vi "nivi.vi"() -> ()   [LabVIEW 2014]
uses:
  <vilib>/Analysis/NI_AALPro.lvlib
panel:
  in  "frequency 4":dbl=10.0 format="%0.2f"
  in  "frequency 3":dbl=10.0 format="%0.2f"
  out "unipolar NRZ 2":dbl[](graph)
  in  "frequency 2":dbl=10.0 format="%0.2f"
  in  "frequency":dbl=10.0 format="%0.2f"
  out "unipolar NRZ":dbl[](graph)
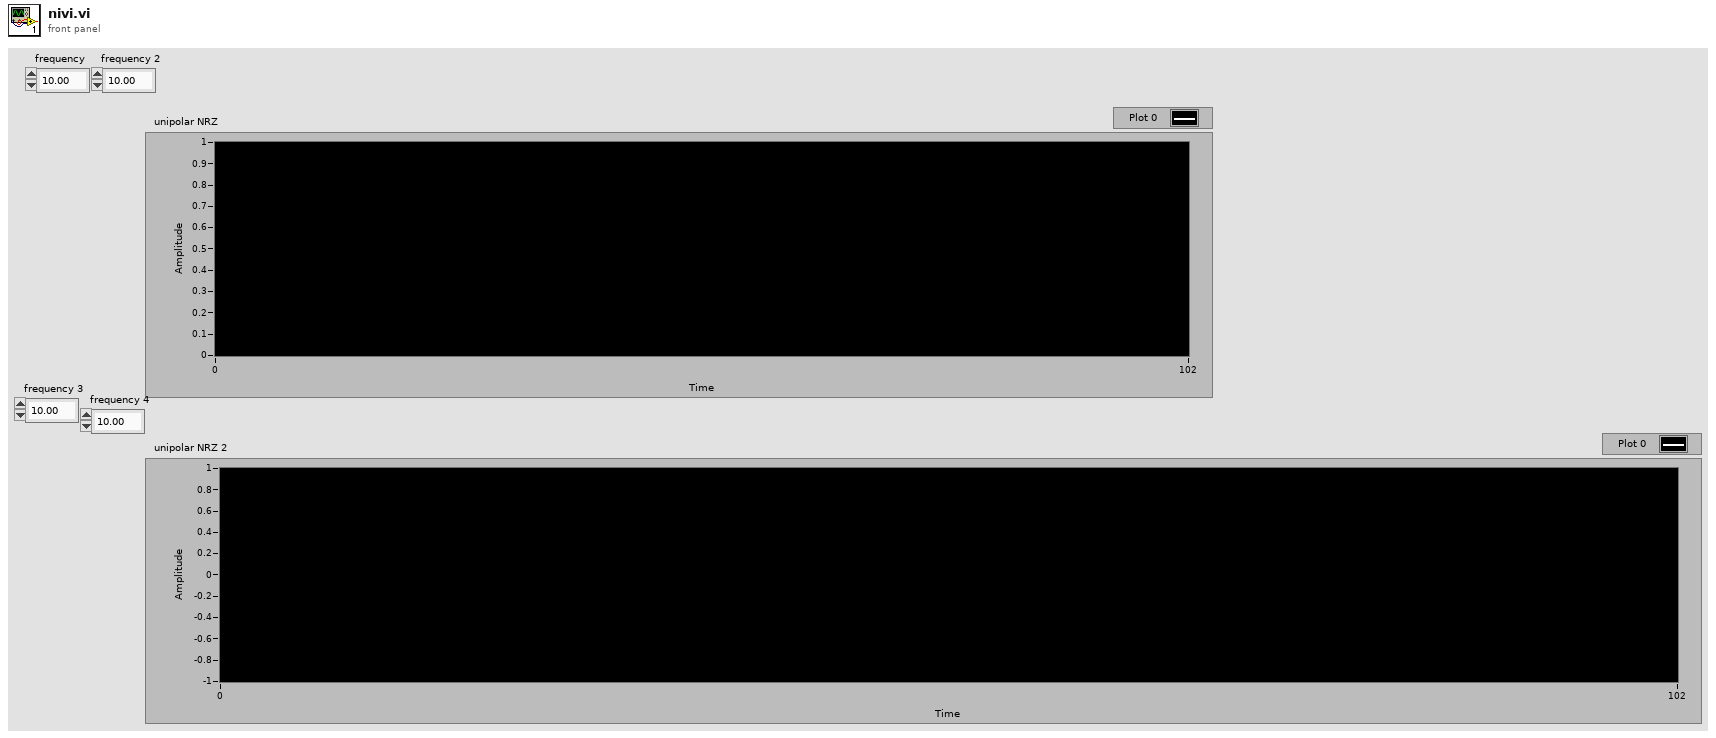
[diagram p1: front panel]
types:
  T1 = enum16{"sine", "cosine", "triangle", "square", "sawtooth", "increasing ramp", "decreasing ramp"}
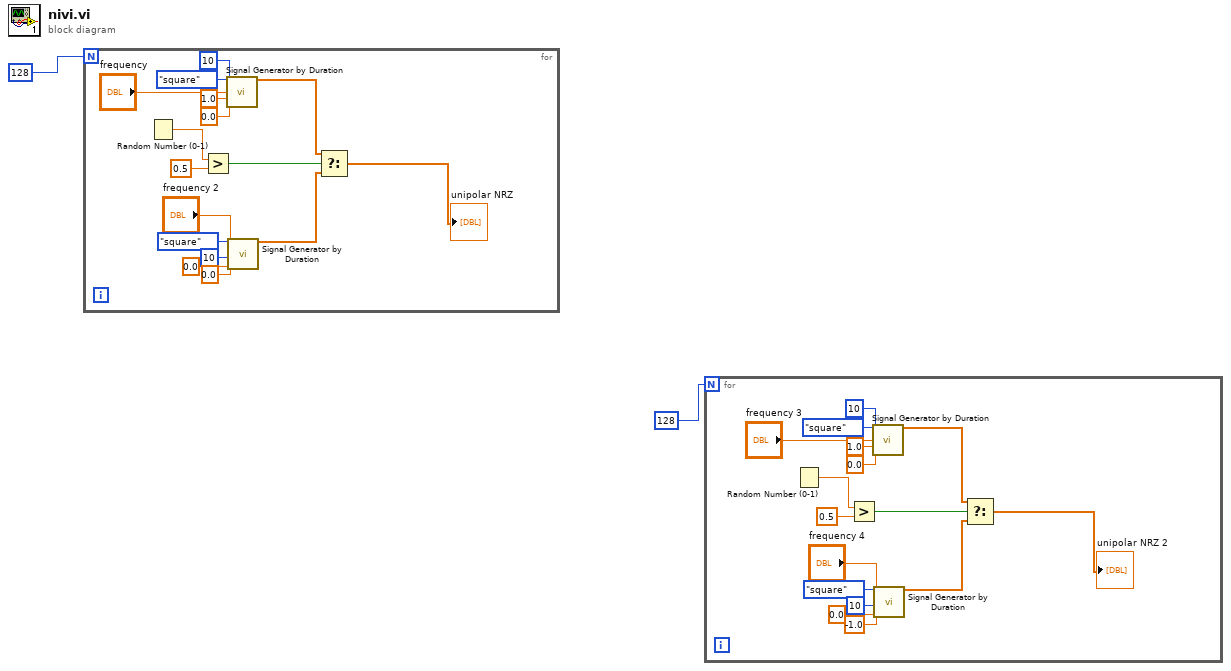
[diagram p0: block diagram]
diagram:
  n1 = for {
    N: 128 -> [_]
    n2 = Random Number (0-1)() -> (number: 0 to 1=w18:dbl)
    n3 = Greater?(x=w18, y=0.5) -> (0:w16:bool)
    n4 = call <vilib>:"Signal Generator by Duration.vi"("signal type"=T1."square", "# of samples"=10, "frequency"="frequency", "amplitude"=1.0, "dc offset"=0.0) -> ("signal"=w15:dbl[])  [unwired: 7 in, 3 out]
    n5 = call <vilib>:"Signal Generator by Duration.vi"("signal type"=T1."square", "# of samples"=10, "frequency"="frequency 2", "amplitude"=0.0, "dc offset"=0.0) -> ("signal"=w14:dbl[])  [unwired: 7 in, 3 out]
    n6 = Select(t=w15, s=w16, f=w14) -> (s? t:f=→"unipolar NRZ":dbl[])
  }
  n7 = for {
    N: 128 -> [_]
    n8 = Random Number (0-1)() -> (number: 0 to 1=w34:dbl)
    n9 = Greater?(x=w34, y=0.5) -> (0:w32:bool)
    n10 = call <vilib>:"Signal Generator by Duration.vi"("signal type"=T1."square", "# of samples"=10, "frequency"="frequency 3", "amplitude"=1.0, "dc offset"=0.0) -> ("signal"=w31:dbl[])  [unwired: 7 in, 3 out]
    n11 = call <vilib>:"Signal Generator by Duration.vi"("signal type"=T1."square", "# of samples"=10, "frequency"="frequency 4", "amplitude"=-1.0, "dc offset"=0.0) -> ("signal"=w30:dbl[])  [unwired: 7 in, 3 out]
    n12 = Select(t=w31, s=w32, f=w30) -> (s? t:f=→"unipolar NRZ 2":dbl[])
  }
